vi "Command processing - 4 wheel omni.vi"(9 "Rotation scaling":dbl=0.5, 10 "Speed (0 to 1)":dbl=0.25, 11 "Command":T1(ring)) -> (0 "Right":dbl, 1 "Left":dbl, 2 "Bottom":dbl, 3 "Top":dbl)   [LabVIEW 2016]
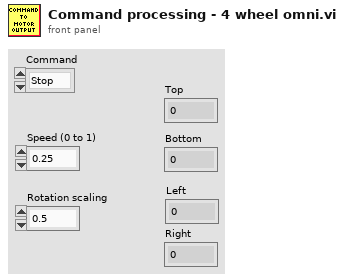
[diagram p1: front panel]
types:
  T1 = enum16{"Stop", "Forward", "Backward", "Left", "Right", "Clockwise", "Anticlockwise"}
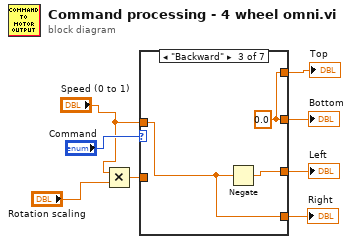
[diagram p0: block diagram]
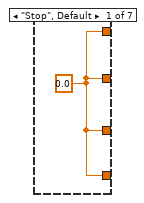
[diagram p2: hidden frame]
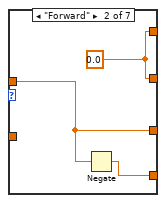
[diagram p3: hidden frame]
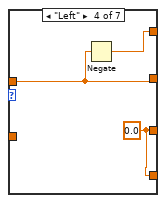
[diagram p4: hidden frame]
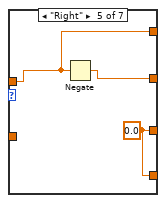
[diagram p5: hidden frame]
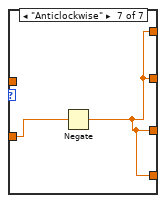
[diagram p7: hidden frame]
diagram:
  n1 = Multiply(x="Speed (0 to 1)", y="Rotation scaling") -> (x*y=w1:dbl)
  n2 = case shown="\"Backward\"" "Command" {
    tunnel: [w9 w12 w13 w18 w20 w22 w23] -> w7
    tunnel: [w9 w12 w13 w17 w21 w22 w23] -> w6
    tunnel: [w9 w11 w15 w16 w19 w22 w23] -> w5
    tunnel: [w9 w10 w14 w16 w19 w22 w23] -> w4
    tunnel: "Speed (0 to 1)" -> [_ w11 w14 w17 w20 _ _]
    tunnel: w1 -> [_ _ _ _ _ w22 w24]
    frame "Stop", Default {
      w9 = 0.0 ("Top")
    }
    frame "Forward" {
      w12 = 0.0 ("Top")
      n3 = Negate(x=w11) -> (-x=w10:dbl)
    }
    frame "Backward" {
      w13 = 0.0 ("Speed (-1 to 1)")
      n4 = Negate(x=w14) -> (-x=w15:dbl)
    }
    frame "Left" {
      w16 = 0.0 ("Speed (-1 to 1)")
      n5 = Negate(x=w17) -> (-x=w18:dbl)
    }
    frame "Right" {
      w19 = 0.0 ("Speed (-1 to 1)")
      n6 = Negate(x=w20) -> (-x=w21:dbl)
    }
    frame "Clockwise" {
    }
    frame "Anticlockwise" {
      n7 = Negate(x=w24) -> (-x=w23:dbl)
    }
  }
  "Top" <- w7
  "Bottom" <- w6
  "Left" <- w5
  "Right" <- w4
